vi "testReadData.vi"() -> ()   [LabVIEW 2025]
panel:
  out "error out 2":errorcluster
  out "error out":errorcluster
  out "read buffer":string
  in  "VISA resource name":refnum<visa-resource-name>
  out "Waveform Chart":u8[](graph)
  in  "Stop":bool
  in  "Start":bool
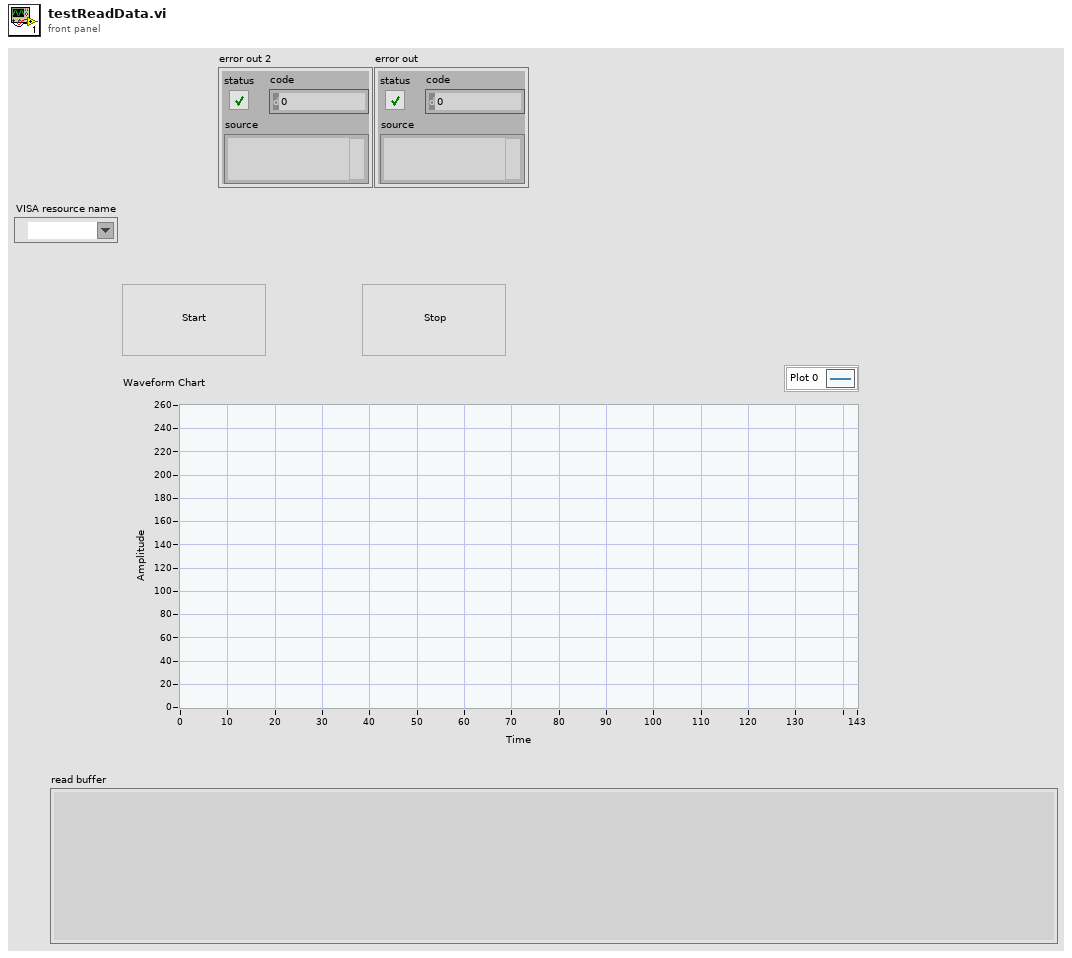
[diagram p1: front panel]
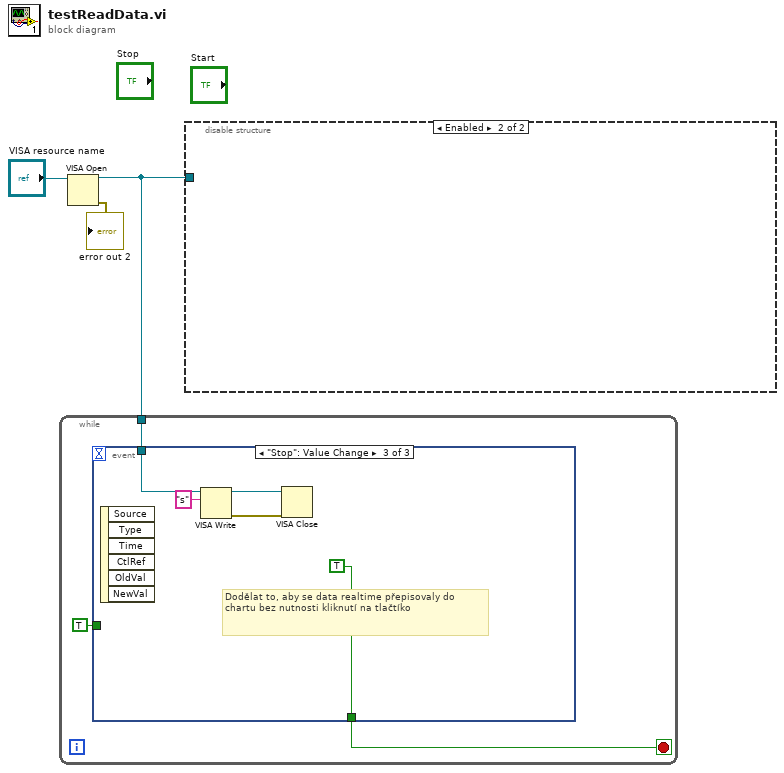
[diagram p0: block diagram]
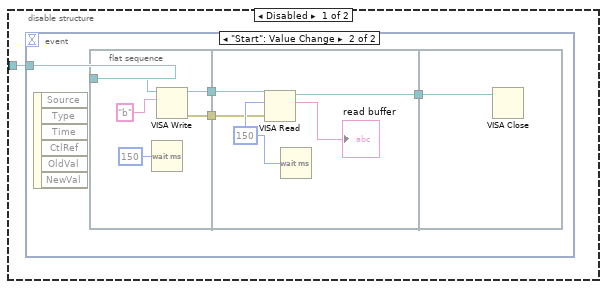
[diagram p2: hidden frame]
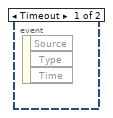
[diagram p3: hidden frame]
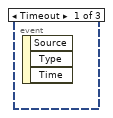
[diagram p4: hidden frame]
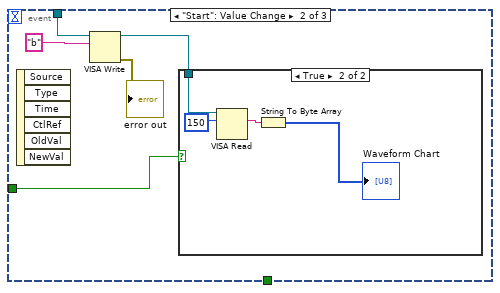
[diagram p5: hidden frame]
diagram:
  n1 = VISA Open(VISA resource name="VISA resource name") -> (VISA resource name=w2:refnum<visa-resource-name>, error out=→"error out 2":errorcluster)  [unwired: 4 in]
  n2 = while {
    tunnel: w2 -> [w6]
    stop <- w5 stop-if-true
    n3 = event shown="[2] \"Stop\": Value Change" {
      selector: _ -> [_ _ _]
      dyn-events: _ -> [_ _ _]
      timeout: _ -> [_ _ _]
      tunnel: w6 -> [_ w11 w20]
      tunnel: [_ _ TRUE] -> w5
      tunnel: TRUE -> [_ w7 _]
      event Timeout {
        n4 = event-data() -> ()  [unwired: 1 in, 3 out]
      }
      event "Start": Value Change {
        n5 = event-data() -> ()  [unwired: 1 in, 6 out]
        n6 = VISA Write(VISA resource name=w11, write buffer="b") -> (VISA resource name out=w9:refnum<visa-resource-name>, error out=→"error out":errorcluster)  [unwired: 1 in, 1 out]
        n7 = case shown="True" w7 {
          tunnel: w9 -> [_ w15]
          frame False {
          }
          frame True {
            n8 = VISA Read(VISA resource name=w15, byte count=u32 150) -> (read buffer=w13:string)  [unwired: 1 in, 3 out]
            n9 = String To Byte Array(string=w13) -> (unsigned byte array=→"Waveform Chart":u8[])
          }
        }
      }
      event "Stop": Value Change {
        # "Dodělat to, aby se data realtime přepisovaly do \nchartu bez nutnosti kliknutí na tlačtíko"
        n10 = event-data() -> ()  [unwired: 1 in, 6 out]
        n11 = VISA Write(VISA resource name=w20, write buffer="s") -> (VISA resource name out=w18:refnum<visa-resource-name>, error out=w17:errorcluster)  [unwired: 1 in, 1 out]
        n12 = VISA Close(VISA resource name=w18, error in (no error)=w17) -> ()  [unwired: 1 out]
      }
    }
  }
  n13 = disable-structure shown="Enabled" {
    disable-tunnel: w2 -> [w21 _]
    frame Disabled {
      n14 = event shown="[1] \"Start\": Value Change" {
        selector: _ -> [_ _]
        dyn-events: _ -> [_ _]
        timeout: _ -> [_ _]
        tunnel: w21 -> [_ w25]
        event Timeout {
          n15 = event-data() -> ()  [unwired: 1 in, 3 out]
        }
        event "Start": Value Change {
          n16 = event-data() -> ()  [unwired: 1 in, 6 out]
          n17 = flat-sequence {
            tunnel: w25 -> [w30]
            tunnel: [w27] -> w24
            tunnel: [w26] -> w23
            tunnel: w24 -> [w33]
            tunnel: w23 -> [w32]
            tunnel: [w31] -> w22
            tunnel: w22 -> [w36]
            frame #0 {
              n18 = Wait (ms)(milliseconds to wait=u32 150) -> ()  [unwired: 1 out]
              n19 = VISA Write(VISA resource name=w30, write buffer="b") -> (VISA resource name out=w27:refnum<visa-resource-name>, error out=w26:errorcluster)  [unwired: 1 in, 1 out]
            }
            frame #1 {
              w34 = u32 150 ("byte count")
              n20 = VISA Read(VISA resource name=w33, byte count=w34, error in (no error)=w32) -> (VISA resource name out=w31:refnum<visa-resource-name>, read buffer=→"read buffer":string)  [unwired: 2 out]
              n21 = Wait (ms)(milliseconds to wait=w34) -> ()  [unwired: 1 out]
            }
            frame #2 {
              n22 = VISA Close(VISA resource name=w36) -> ()  [unwired: 1 in, 1 out]
            }
          }
        }
      }
    }
    frame Enabled {
    }
  }
